vi "User2Formal setting.vi"(10 "Setting User Input":T5 {"Zoom (V)" scale=0.0..1.0; "X Pos." scale=-2.0..2.0; "Y Pos." scale=-2.0..2.0}, 11 "IntensityGraph输入":refnum<vi>) -> (0 "错误输出":errorcluster, 2 "Image 2":T4, 3 "Status":T1 {"Setting"."X Pos." scale=-2.0..2.0; "Setting"."Y Pos." scale=-2.0..2.0})   [LabVIEW 2013]
uses:
  Setting-User input.ctl
  imaging/Image.ctl
  init-status.ctl
  Setting.ctl
  event-package.ctl
  Event1.ctl
  data-package.ctl
  Event.ctl
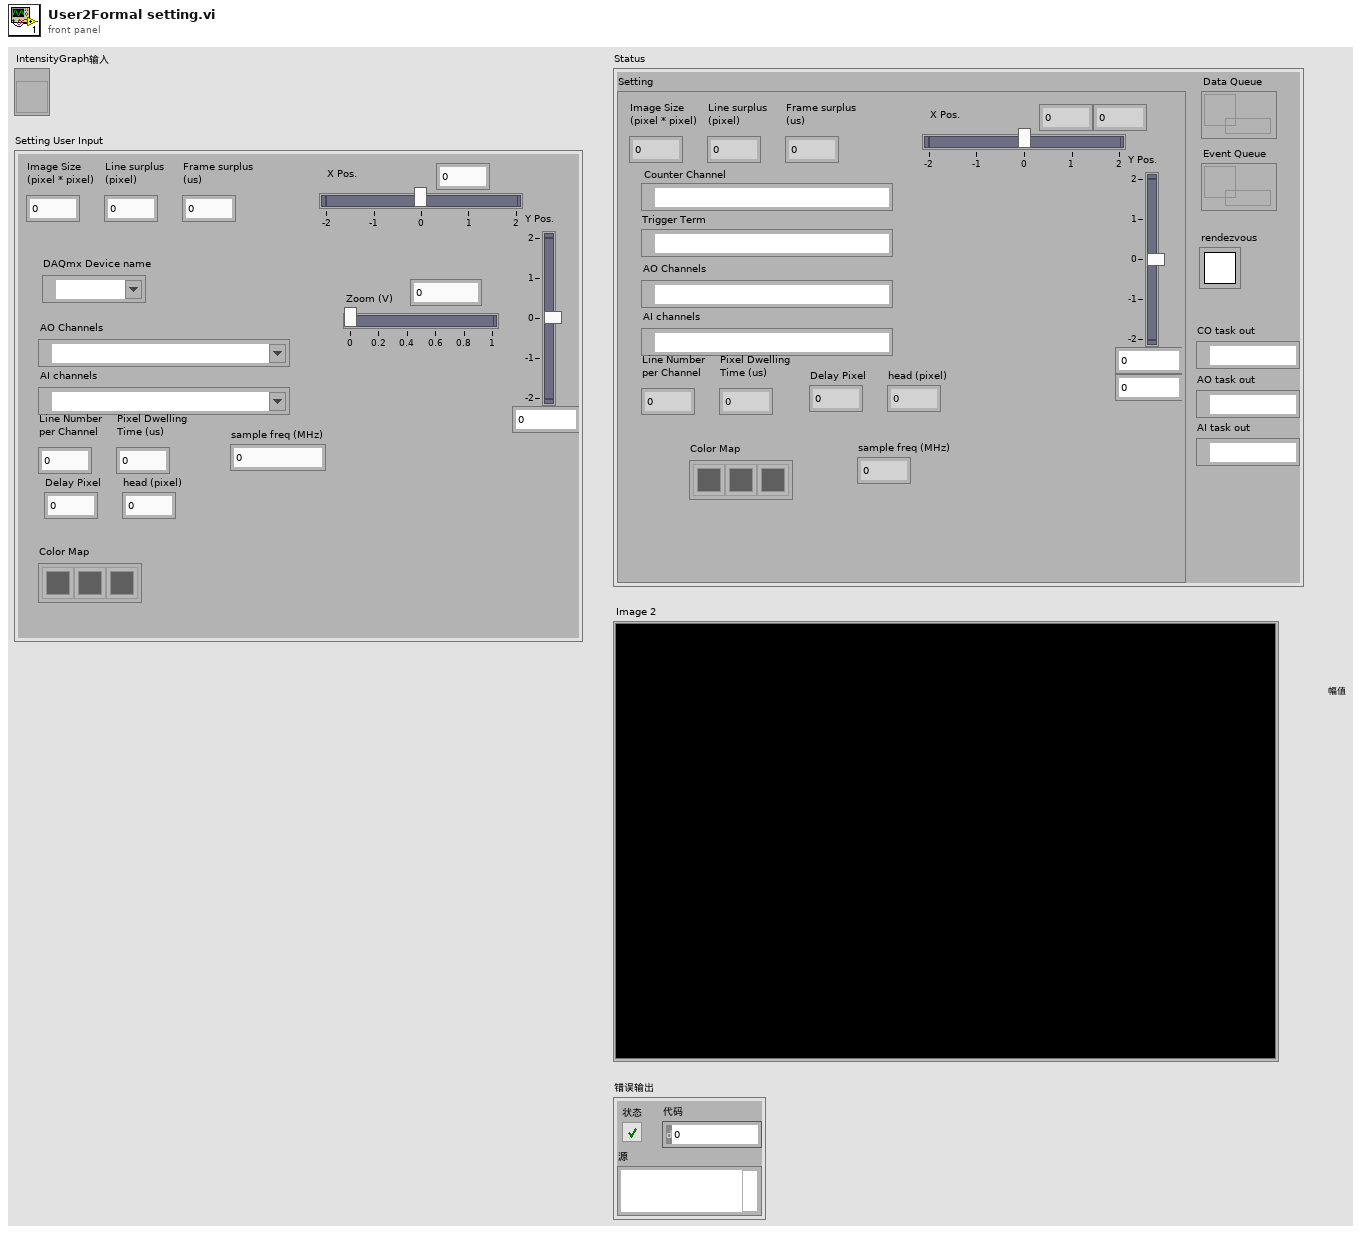
[diagram p1: front panel]
types:
  T1 = typedef "init-status.ctl" = cluster{"Setting":T2, "Event Queue":refnum<queue>, "Data Queue":refnum<queue>, "rendezvous":T3, "CO task out":refnum<k21>, "AO task out":refnum<k21>, "AI task out":refnum<k21>}
  T2 = typedef "Setting.ctl" = cluster{"Image Size\n(pixel * pixel)":i32, "Counter Channel":tag, "Trigger Term":tag, "AO Channels":tag, "Y Pos.":cluster{dbl, dbl}, "X Pos.":cluster{dbl, dbl}, "Line surplus\n(pixel)":i32, "Frame surplus\n(us)":i32, "AI channels":tag, "Line Number\nper Channel":i32, "Delay Pixel":i32, "Pixel Dwelling\nTime (us)":i32, "Color Map":u32[], "head (pixel)":i32, "sample freq (MHz)":dbl}
  T3 = typedef "Rendezvous RefNum" = refnum<k1>
  T4 = typedef "Image.ctl" = dbl[][]
  T5 = typedef "Setting-User input.ctl" = cluster{"Image Size\n(pixel * pixel)":i32, "AO Channels":tag, "Y Pos.":dbl, "X Pos.":dbl, "Line surplus\n(pixel)":i32, "Frame surplus\n(us)":i32, "AI channels":tag, "Line Number\nper Channel":i32, "Delay Pixel":i32, "Pixel Dwelling\nTime (us)":i32, "Color Map":u32[], "head (pixel)":i32, "Zoom (V)":dbl, "DAQmx Device name":tag, "sample freq (MHz)":dbl}
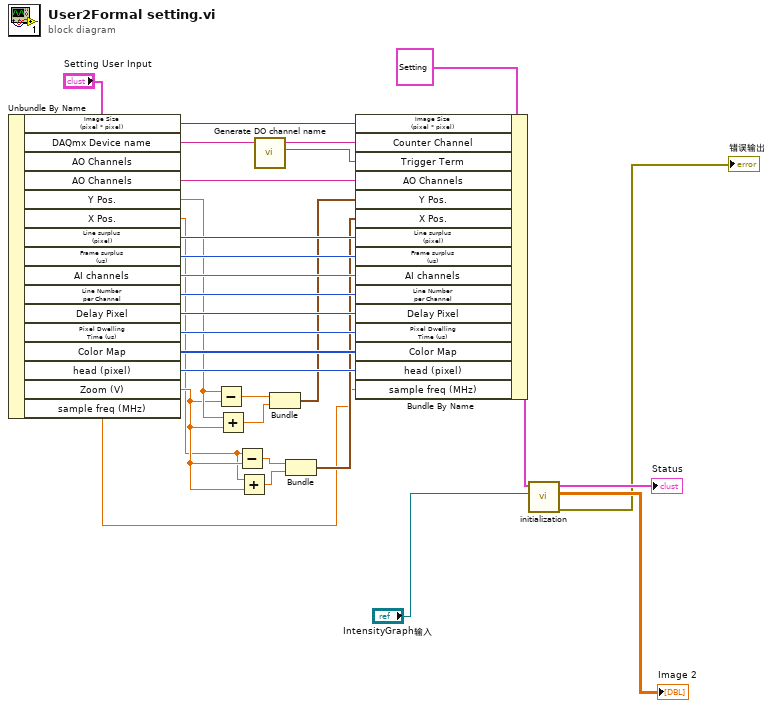
[diagram p0: block diagram]
diagram:
  n1 = Unbundle By Name("Setting User Input") -> ("Image Size\n(pixel * pixel)"=w22:i32, "DAQmx Device name"=w2:tag, "AO Channels"=w21:tag, "Y Pos."=w13:dbl, "X Pos."=w8:dbl, "Line surplus\n(pixel)"=w20:i32, "Frame surplus\n(us)"=w19:i32, "AI channels"=w18:tag, "Line Number\nper Channel"=w17:i32, "Delay Pixel"=w16:i32, "Pixel Dwelling\nTime (us)"=w15:i32, "Color Map"=w14:u32[], "head (pixel)"=w23:i32, "Zoom (V)"=w9:dbl, "sample freq (MHz)"=w1:dbl)  [unwired: 1 out]
  n2 = Subtract(x=w13, y=w9) -> (x-y=w12:dbl)
  n3 = Add(x=w13, y=w9) -> (x+y=w11:dbl)
  n4 = Subtract(x=w8, y=w9) -> (x-y=w7:dbl)
  n5 = Add(x=w8, y=w9) -> (x+y=w6:dbl)
  n6 = call "Generate DO channel name.vi"("DAQmx Device name"=w2) -> ("Trigger Term"=w3:tag, "Counter Channel"=w4:tag)  [unwired: 9 in]
  n7 = Bundle(w12, w11) -> (w10:cluster{dbl, dbl})  [unwired: 1 in]
  n8 = Bundle(w7, w6) -> (w5:cluster{dbl, dbl})  [unwired: 1 in]
  n9 = Bundle By Name(cluster=T2 {"Image Size\n(pixel * pixel)"=0, "Counter Channel"="", "Trigger Term"="", "AO Channels"="", "Y Pos."={0.0, 0.0}, "X Pos."={0.0, 0.0}, "Line surplus\n(pixel)"=0, "Frame surplus\n(us)"=0, "AI channels"="", "Line Number\nper Channel"=0, "Delay Pixel"=0, "Pixel Dwelling\nTime (us)"=0, "Color Map"=[], "head (pixel)"=0, "sample freq (MHz)"=0.0} ("Setting"), "Image Size\n(pixel * pixel)"=w22, "Counter Channel"=w4, "Trigger Term"=w3, "AO Channels"=w21, "Y Pos."=w10, "X Pos."=w5, "Line surplus\n(pixel)"=w20, "Frame surplus\n(us)"=w19, "AI channels"=w18, "Line Number\nper Channel"=w17, "Delay Pixel"=w16, "Pixel Dwelling\nTime (us)"=w15, "Color Map"=w14, "head (pixel)"=w23, "sample freq (MHz)"=w1) -> (w25:T2)
  n10 = call "initialization.vi"("IntensityGraph输入"="IntensityGraph输入", "Setting"=w25) -> ("error out"=→"错误输出":errorcluster, "Image"=→"Image 2":T4, "Status"=→"Status":T1)  [unwired: 7 in]
